vi "Sort system control metadata.vi"(0 "reference in":refnum<class "metadata.lvclass">, 5 "error in (no error)":errorcluster) -> (14 "reference out":refnum<class "metadata.lvclass">, 16 "System control cluster":T1, 19 "error out":errorcluster)   [LabVIEW 2019]
uses:
  metadata.lvclass
  System control parameters.ctl
panel:
  out "Array":string[](array[string])
  out "Array 2":i32[](array[numeric])
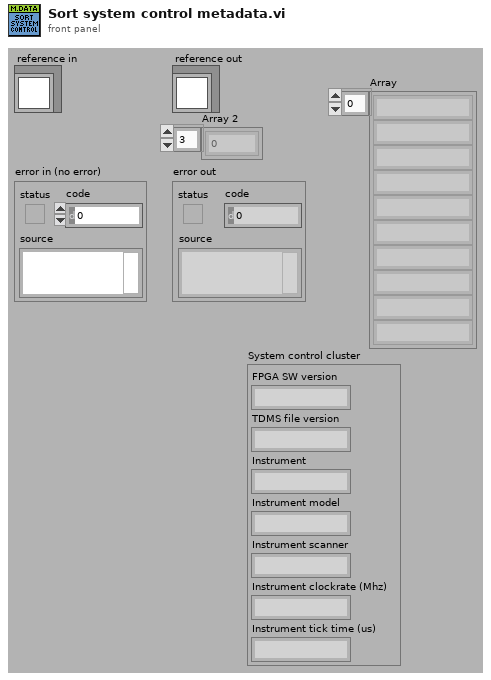
[diagram p1: front panel]
types:
  T1 = typedef "metadata.lvclass/System control parameters.ctl" = cluster{"FPGA SW version":string, "TDMS file version":string, "Instrument":string, "Instrument model":string, "Instrument scanner":string, "Instrument clockrate (Mhz)":string, "Instrument tick time (us)":string}
  T2 = typedef "metadata.lvclass/ObjectAttributesRef.ctl" = refnum<data-value>
  T3 = typedef "metadata.lvclass/ObjectAttributes.ctl" = cluster{"MyAttribute":dbl, "System Control":T1, "file info":T4, "Sample info":T5, "Cantilever info":T6, "XYZ piezos":T7, "Mapping":T8, "Fcurve segment":T9[], "Fast fpga segment":T11, "Chirp":T12, "precision (6)":i16, "width (-)":i16, "Metadata":T13, "config filepath":path, "Section names []":string[], "Property names []":string[], "nb elements":u16}
  T4 = typedef "metadata.lvclass/File info parameters.ctl" = cluster{"Time Stamp":timestamp, "Filename":string, "Filepath":path, "User":string, "Experiment_name":string, "Curve_id":string, "number_segments":u8, "number_consecutive_scans":u32}
  T5 = typedef "metadata.lvclass/Sample info parameters.ctl" = cluster{"Sample name":string, "Sample species":string}
  T6 = typedef "metadata.lvclass/Cantilever info parameters.ctl" = cluster{"spring constant calib method":string, "invOLS calib method":string, "thermal calib deflection channel":string, "model":string, "shape":string, "tip geometry":string, "Laser sum (V)":dbl, "Laser power (mA)":dbl, "invOLS_(nm/V)":dbl, "spring constant nominal (N/m)":dbl, "spring constant calib (N/m)":dbl, "resosnance frequency air calib (Hz)":dbl, "resosnance frequency calib (Hz)":dbl, "quality factor":dbl, "Acoefficident_GCI_(nN.s^1.3/m)":dbl, "half angle (deg)":dbl, "tip radius (m)":dbl, "tip height (m)":dbl, "system mount angle (deg)":dbl}
  T7 = typedef "metadata.lvclass/XYZ piezos parameters.ctl" = cluster{"X stage piezo sensitivity (nm/V)":dbl, "X stage piezo gain":dbl, "X velocity (V/tick)":dbl, "X closed loop":bool, "Y stage piezo sensitivity (nm/V)":dbl, "Y stage piezo gain":dbl, "Y velocity (V/tick)":dbl, "Y closed loop":bool, "Z stage piezo sensitivity (nm/V)":dbl, "Z stage piezo gain":dbl, "Z closed loop":bool, "X position (V)":dbl, "Y position (V)":dbl}
  T8 = typedef "metadata.lvclass/Mapping parameters.ctl" = cluster{"Mapping":bool, "index":u16, "position row":u16, "position column":u16, "next position row":i16, "next position column":i16, "X initial position (V)":dbl, "Y initial position (V)":dbl, "X step size (V)":dbl, "Y step size (V)":dbl}
  T9 = typedef "metadata.lvclass/Fcurve segment.ctl" = cluster{"type":T10, "fast_fpga_trigger":bool, "nb":u8, "duration (ticks)":i64, "nb points":i32, "sampling rate (S/s)":u32, "Zpiezo control out":string, "initial deflection (V)":dbl, "relative setpoint":bool, "setpoint on":bool, "setpoint (V)":dbl, "setpoint trigger channel":string, "velocity (V/tick)":dbl, "Z position setpoint trigger (V)":dbl, "Z retract length (V)":dbl, "dec factor":u32}
  T10 = typedef "metadata.lvclass/Segment type--combobox.ctl" = string
  T11 = typedef "metadata.lvclass/fast fpga segment parameters.ctl" = cluster{"Fast start time trigger":timestamp, "nb_points":u32, "sampling_rate_(S/s)":u32, "duration_(ticks)":u32}
  T12 = typedef "metadata.lvclass/Chirp added parameters.ctl" = cluster{"f start (Hz)":dbl, "f end (Hz)":dbl, "Sweep type":string}
  T13 = typedef "metadata.lvclass/Metadata output --cluster.ctl" = cluster{"Property Names":string[], "Property Values":variant[]}
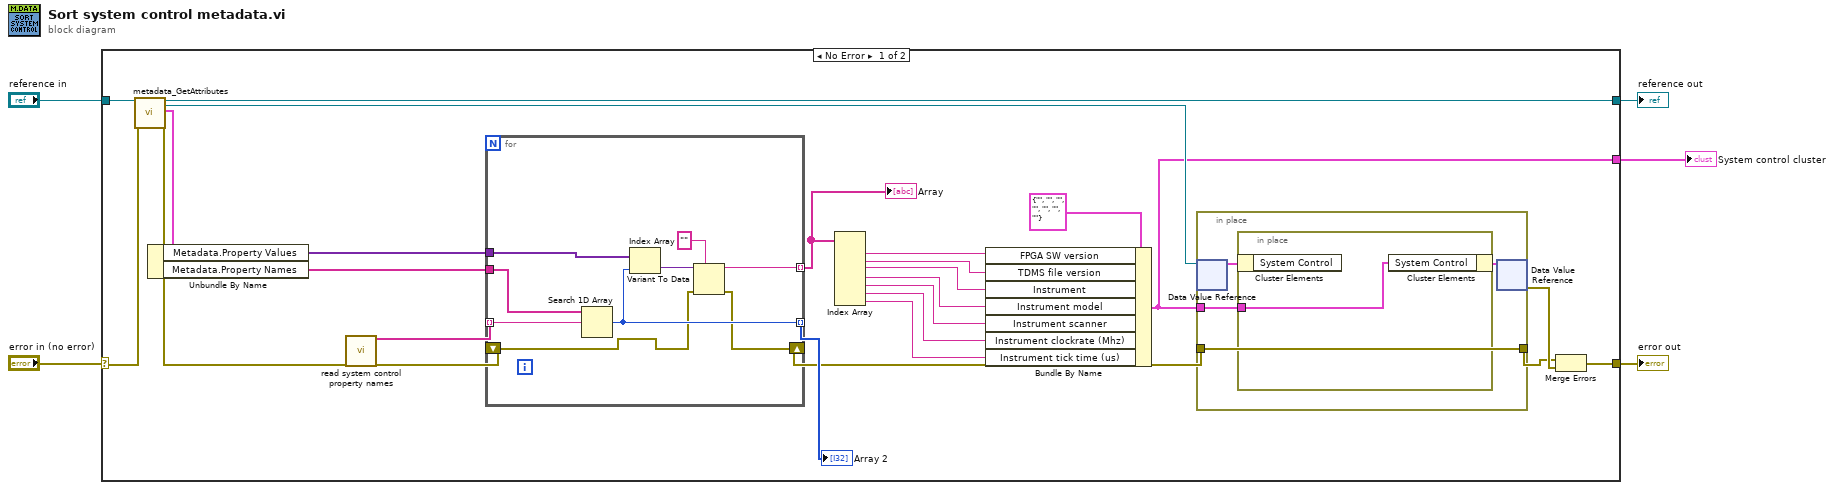
[diagram p0: block diagram]
diagram:
  n1 = case shown="No Error" "error in (no error)" {
    selector: "error in (no error)" -> [w26 w46]
    tunnel: [w30 w46] -> w4
    tunnel: [w25 w45] -> w2
    tunnel: "reference in" -> [w27 w45]
    tunnel: [w6 _] -> w1
    frame No Error {
      n2 = call "metadata_GetAttributes.vi"("reference in"=w27, "error in (no error)"=w26) -> ("reference out"=w25:refnum<class "metadata.lvclass">, "attributes ref"=w24:T2, "attributes"=w23:T3, "error out"=w22:errorcluster)  [unwired: 14 in]
      n3 = Unbundle By Name(w23) -> ("Metadata.Property Values"=w16:variant[], "Metadata.Property Names"=w21:string[])
      n4 = call "read system control property names.vi"("error in (no error)"=w22) -> ("System control"=w20:string[], "error out"=w17:errorcluster)  [unwired: 17 in]
      n5 = for {
        tunnel: w20 -> [w39] mode=indexing
        tunnel: [w36] -> w19 mode=indexing
        shift-right: [w32] -> w18
        shift-left: w17 -> [w33]
        tunnel: w21 -> [w38]
        tunnel: w16 -> [w37]
        tunnel: [w34] -> w14 mode=indexing
        n6 = Search 1D Array(1D array=w38, element=w39) -> (index of element=w36:i32)  [unwired: 1 in]
        n7 = Index Array(array=w37, index=w36) -> (element=w35:variant)
        n8 = Variant To Data(error in=w33, type="", Variant=w35) -> (data=w34:string, error out=w32:errorcluster)
      }
      "Array 2" <- w19
      "Array" <- w14
      n9 = Index Array(array=w14) -> (element #1=w13:string, element #2=w12:string, element #3=w11:string, element #4=w10:string, element #5=w9:string, element #6=w8:string, element #7=w7:string)  [unwired: 7 in]
      n10 = Bundle By Name(cluster=T1 {"FPGA SW version"="", "TDMS file version"="", "Instrument"="", "Instrument model"="", "Instrument scanner"="", "Instrument clockrate (Mhz)"="", "Instrument tick time (us)"=""} ("System Control"), "FPGA SW version"=w13, "TDMS file version"=w12, "Instrument"=w11, "Instrument model"=w10, "Instrument scanner"=w9, "Instrument clockrate (Mhz)"=w8, "Instrument tick time (us)"=w7) -> (w6:T1)
      n11 = in-place {
        in-place-border: w18 -> [w41]
        in-place-border: [w41] -> w28
        in-place-border: w6 -> [w40]
        n12 = in-place-dvr #1(w24) -> (w42:T3)  [unwired: 1 out]
        n13 = in-place {
          in-place-border: w40 -> [w44]
          n14 = in-place-cluster #2(w42) -> ()  [unwired: 1 out]
          n15 = in-place-cluster #2("System Control"=w44) -> (w43:T3)
        }
        n16 = in-place-dvr #1(w43) -> (w29:errorcluster)  [unwired: 1 out]
      }
      n17 = Merge Errors(w28, w29) -> (w30:errorcluster)
    }
    frame Error {
    }
  }
  "error out" <- w4
  "reference out" <- w2
  "System control cluster" <- w1
